vi "Send initalize request msg.vi"(0 "Trigger Timeout (10000000)":dbl=1000.0 format="%#_13g", 1 "Message Enqueuer in":refnum<class "Message Enqueuer.lvclass">, 2 "Control cluster":T2={"Number of points"=816000.0, "Input Range"=10000, "Trigger Level"=29, "Trigger source"=TRUE} {"Trigger Level" min=-100 max=100 step=1 scale=-100.0..100.0; "Input Range" items=["+/- 5 V"=10000, "+/- 2 V"=4000, "+/- 1 V"=2000, "+/- 500 mV"=1000, "+/- 200 mV"=400, "+/- 100 mV"=200]; "Number of points" min=160.0 step=160.0}, 3 "error in (no error)":errorcluster, 4 "Message Priority (Normal)":T1=enum."Normal") -> (7 "Message Enqueuer out":refnum<class "Message Enqueuer.lvclass">, 10 "error out":errorcluster)   [LabVIEW 2015, in "Initialize request msg.lvclass"]
uses:
  Initialize request msg.lvclass
  <vilib>/ActorFramework/Message Enqueuer/Message Enqueuer.lvclass
  <vilib>/ActorFramework/Message Enqueuer/Message Priority.ctl
  Initialize request msg.lvclass/Initialize request msg.ctl
  <vilib>/ActorFramework/Message Enqueuer/Message Enqueuer.lvclass/Message Enqueuer.ctl
  <vilib>/ActorFramework/Message Priority Queue/Priority Enqueue.vi
panel:
  in  "Initialize request msg in":refnum<class "Initialize request msg.lvclass">
  # "Basic Card Controlls"
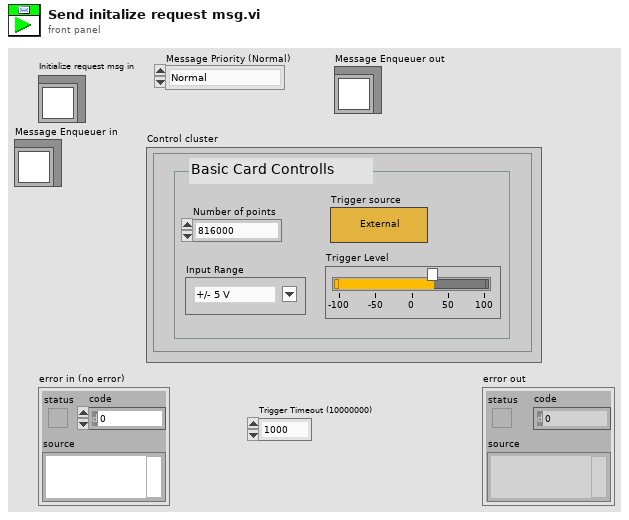
[diagram p1: front panel]
types:
  T1 = typedef "Actor Framework.lvlib/Message Enqueuer.lvclass/Message Priority.ctl" = enum16{"Low", "Normal", "High"}
  T2 = cluster{"Number of points":dbl, "Input Range":u32, "Trigger Level":i32, "Trigger source":bool}
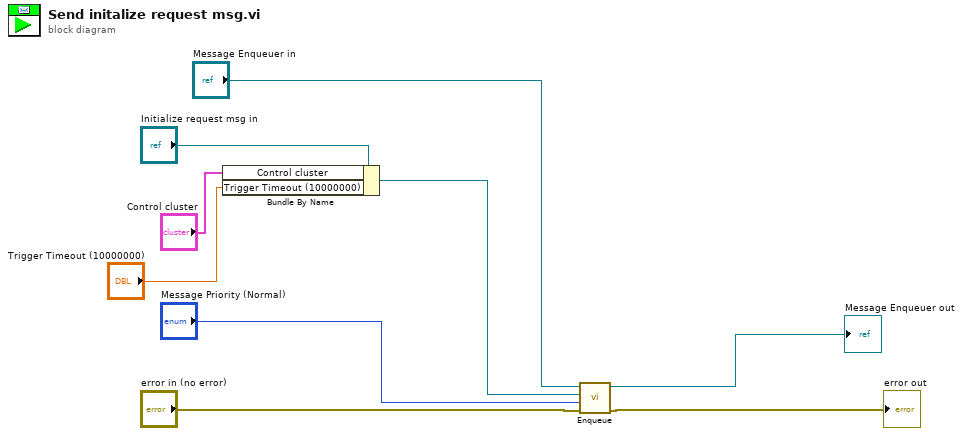
[diagram p0: block diagram]
diagram:
  n1 = Bundle By Name(cluster="Initialize request msg in", "Control cluster"="Control cluster", "Trigger Timeout (10000000)"="Trigger Timeout (10000000)") -> (w5:refnum<class "Initialize request msg.lvclass">)
  n2 = call <vilib>:"Enqueue.vi"("error in (no error)"="error in (no error)", "Message Priority (Normal)"="Message Priority (Normal)", "Message"=w5, "Message Enqueuer in"="Message Enqueuer in") -> ("error out"=→"error out":errorcluster, "Message Enqueuer out"=→"Message Enqueuer out":refnum<class "Message Enqueuer.lvclass">)  [unwired: 6 in]
